vi "Defender.vi"(0 "Field defense":dbl[](array[numeric]), 1 "IA State Input 2":T1, 3 "N atacantes":u32[](array[numeric]), 4 "balls":T4[](array[typedef]), 5 "total de \ndefensores":i32, 6 "geometry":T5, 7 "Defensores":u32[](array[numeric]), 8 "Enemy Robots":T2, 9 "Total de n\natacantes":i32, 10 "Our Robots":T2, 11 "command\nenum":T7) -> (2 "output cluster":T2)   [LabVIEW 2016]
uses:
  Core/AI Robot.ctl
  Functions Enum.ctl
  Command Enum.ctl
  Core/Field Size.ctl
  Core/AI Ball.ctl
  Core/AI Input.ctl
  Core/AI Judge.ctl
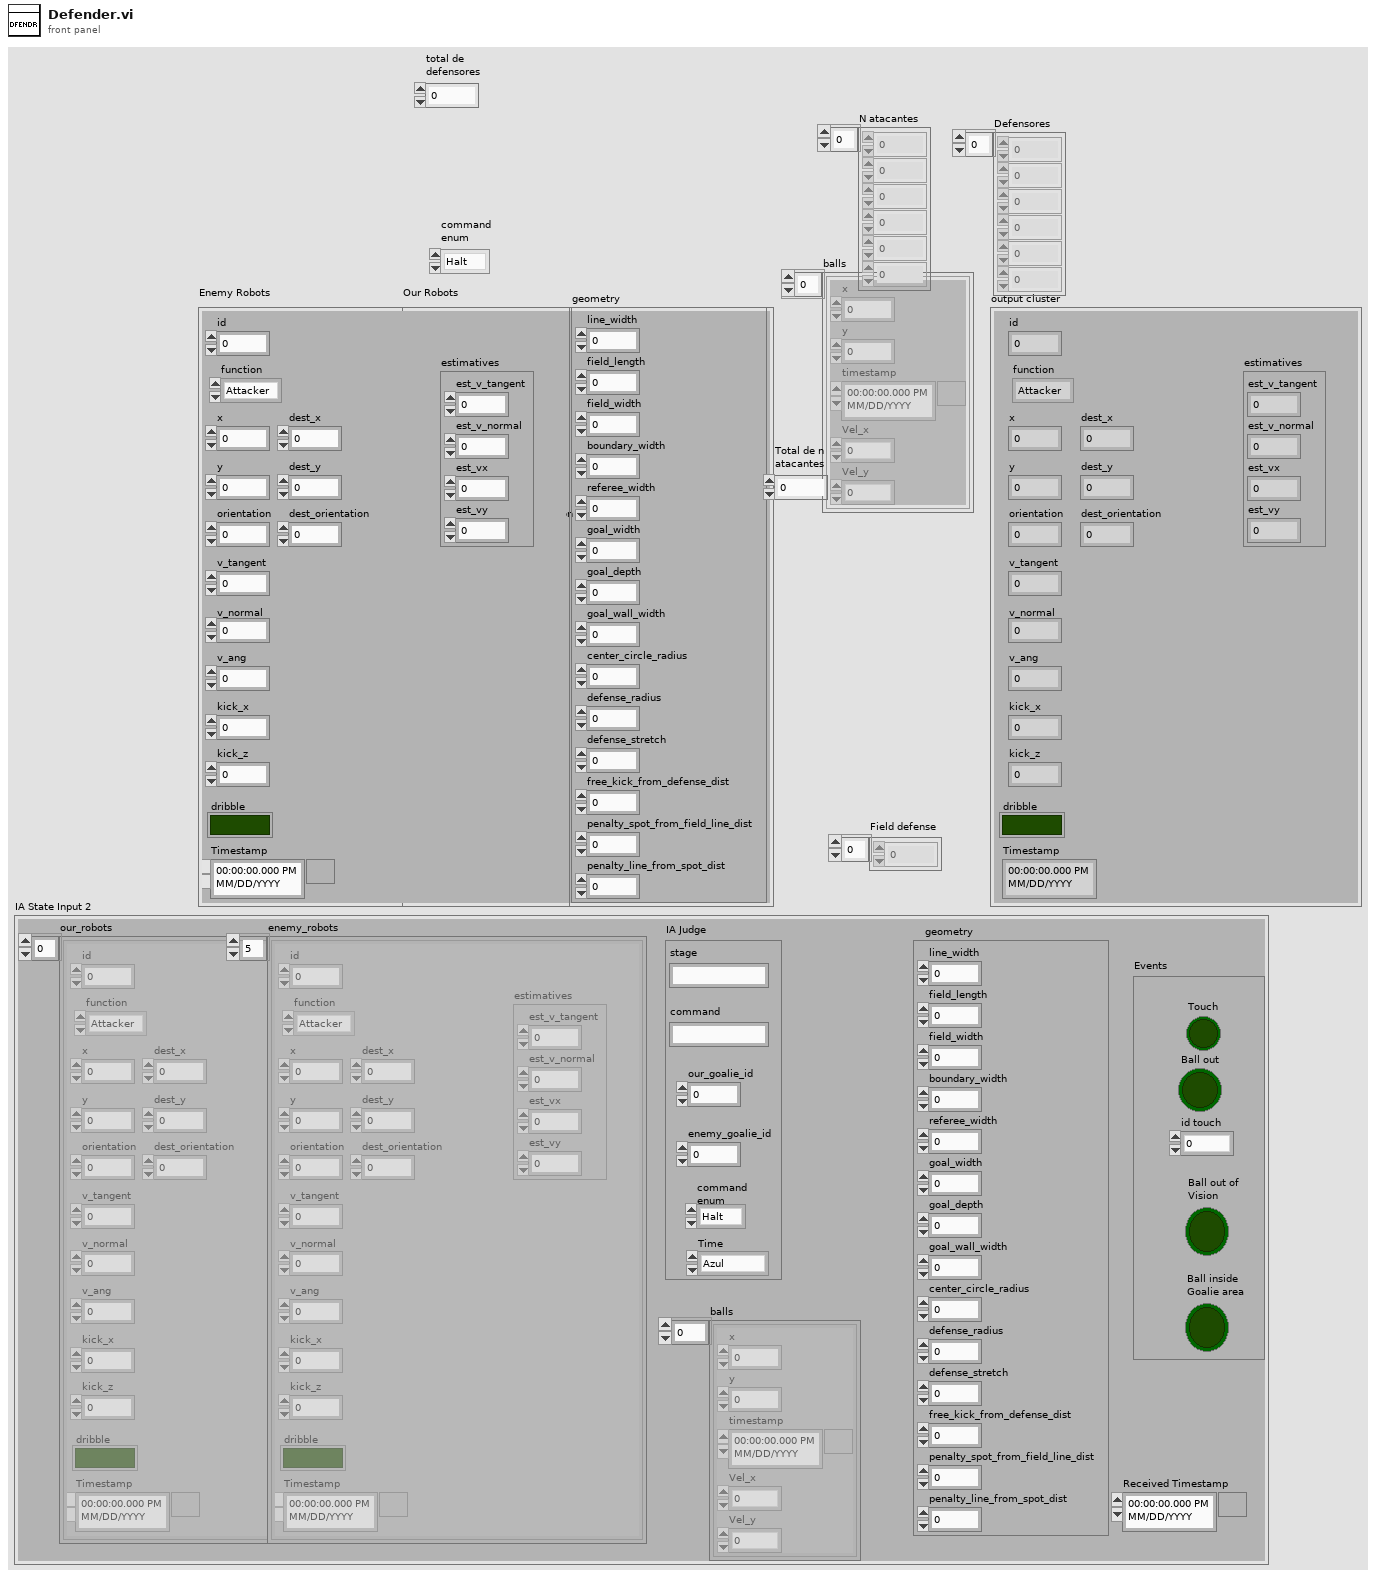
[diagram p1: front panel]
types:
  T1 = typedef "AI Input.ctl" = cluster{"our_robots":T2[], "enemy_robots":T2[], "balls":T4[], "geometry":T5, "IA Judge":T6, "Received Timestamp":timestamp, "Events":cluster{"Touch":bool, "Ball out":bool, "id touch":dbl, "Ball out of \nVision":bool, "Ball inside \nGoalie area":bool}}
  T2 = typedef "AI Robot.ctl" = cluster{"id":u32, "function":T3, "x":dbl, "y":dbl, "orientation":dbl, "v_tangent":dbl, "v_normal":dbl, "v_ang":dbl, "kick_x":dbl, "kick_z":dbl, "dribble":bool, "Timestamp":timestamp, "dest_x":dbl, "dest_y":dbl, "dest_orientation":dbl, "estimatives":cluster{"est_v_tangent":dbl, "est_v_normal":dbl, "est_vx":dbl, "est_vy":dbl}}
  T3 = typedef "Functions Enum.ctl" = enum16{"Attacker", "Goalie", "Defender", "Striker", "Goto 0", "Dummy", "ZigZag"}
  T4 = typedef "AI Ball.ctl" = cluster{"x":dbl, "y":dbl, "timestamp":timestamp, "Vel_x":dbl, "Vel_y":dbl}
  T5 = typedef "Field Size.ctl" = cluster{"line_width":u32, "field_length":u32, "field_width":u32, "boundary_width":u32, "referee_width":u32, "goal_width":u32, "goal_depth":u32, "goal_wall_width":u32, "center_circle_radius":u32, "defense_radius":u32, "defense_stretch":u32, "free_kick_from_defense_dist":u32, "penalty_spot_from_field_line_dist":u32, "penalty_line_from_spot_dist":u32}
  T6 = typedef "AI Judge.ctl" = cluster{"stage":string, "command":string, "our_goalie_id":dbl, "enemy_goalie_id":dbl, "command\nenum":T7, "Time":enum16{"Azul", "Amarelo"}}
  T7 = typedef "Command Enum.ctl" = enum16{"Halt", "Stop", "Force Start", "PKA Normal Start", "Prepare Kickoff Ally", "PKE Normal Start", "Prepare Kickoff Enemy", "Prepare Penalty Ally", "PPA Normal Start", "Prepare Penalty Enemy", "PPE Normal Start", "Direct Free Enemy", "Direct Free Ally", "Indirect Free Enemy", "Indirect Free Ally", "Timeout Enemy", "Timeout Ally", "Goal Enemy", "Goal Ally", "Ball Placement Enemy", "Ball Placement Ally", "None"}
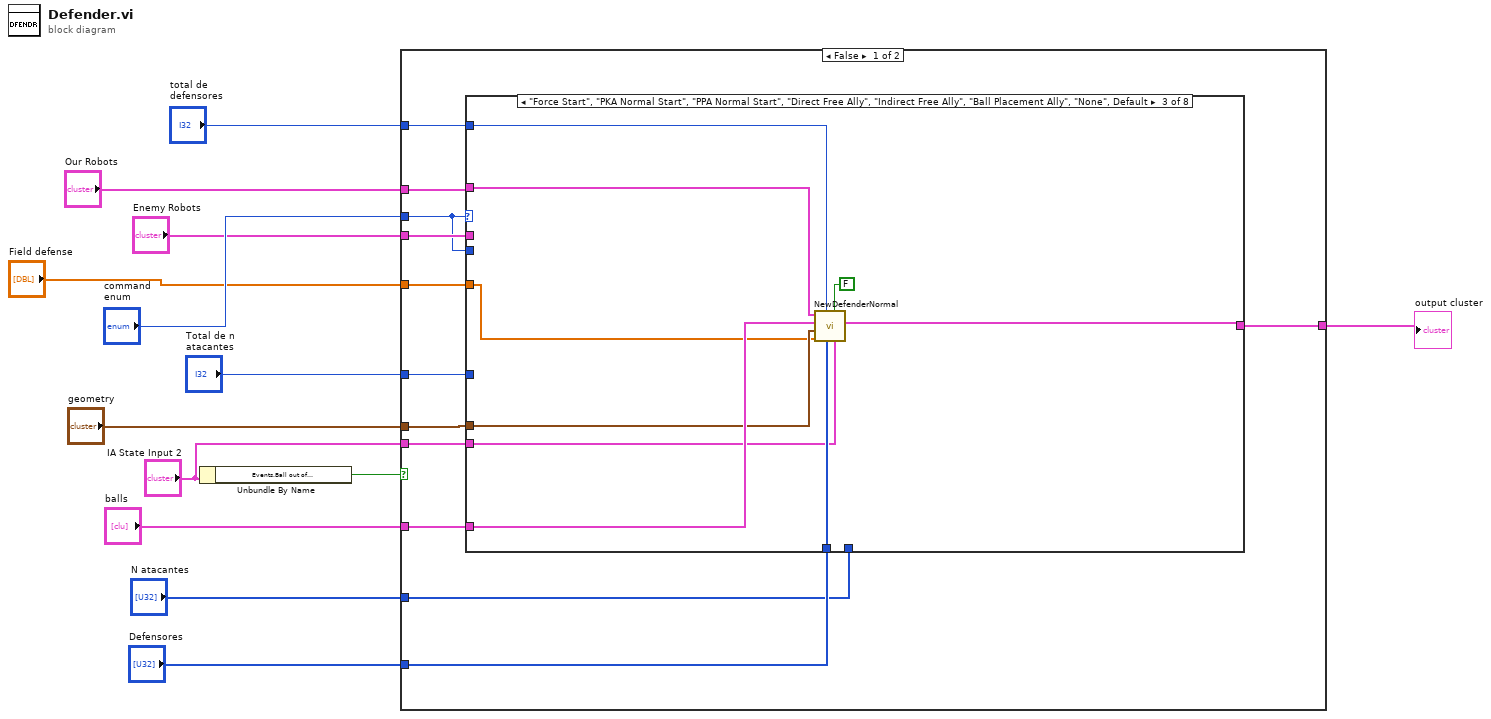
[diagram p0: block diagram]
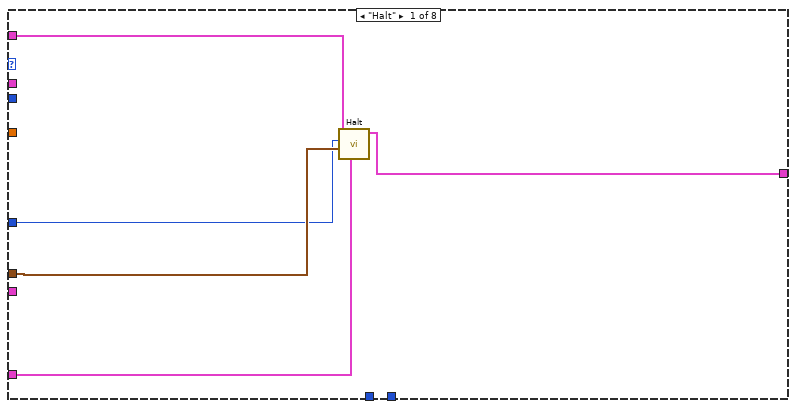
[diagram p2: hidden frame]
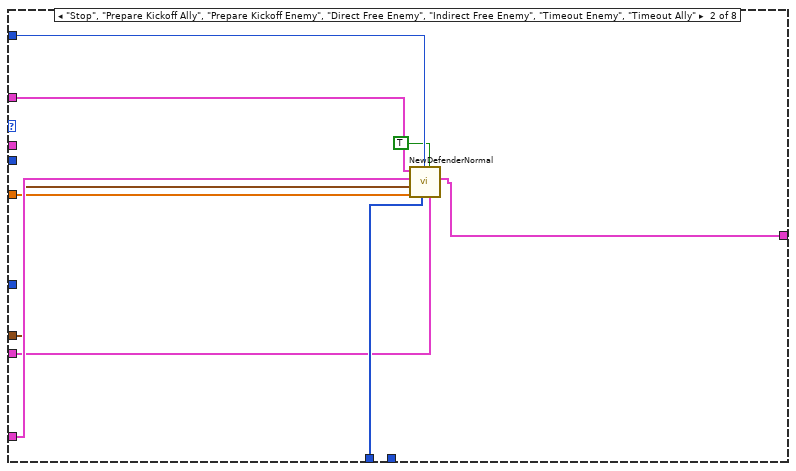
[diagram p3: hidden frame]
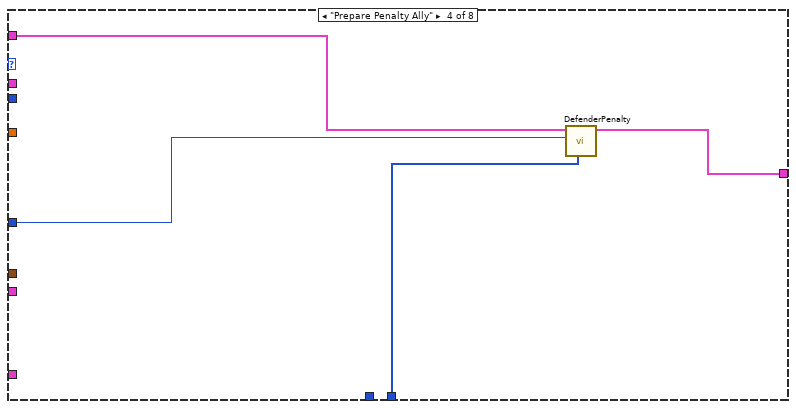
[diagram p4: hidden frame]
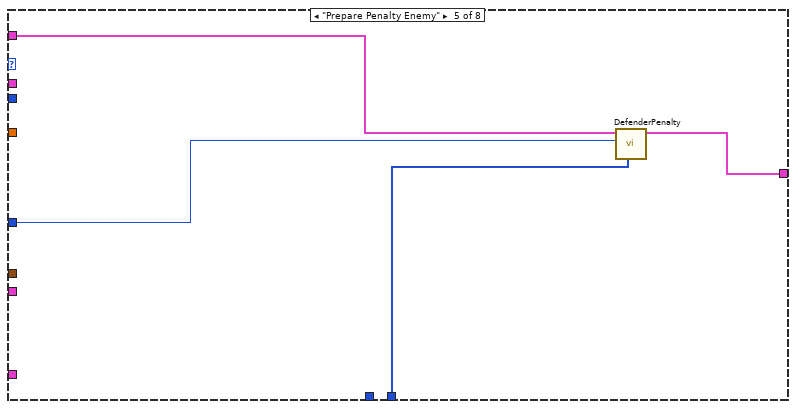
[diagram p5: hidden frame]
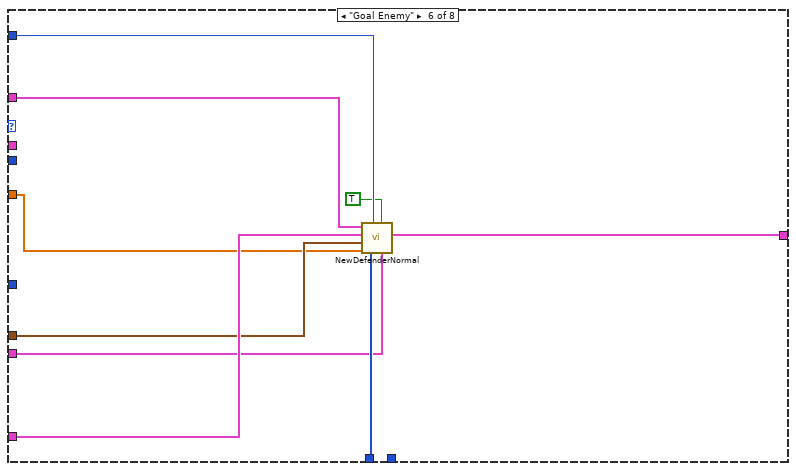
[diagram p6: hidden frame]
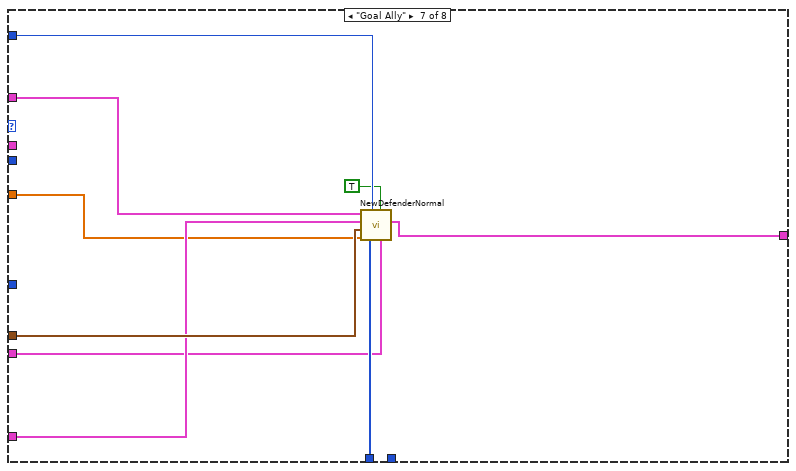
[diagram p7: hidden frame]
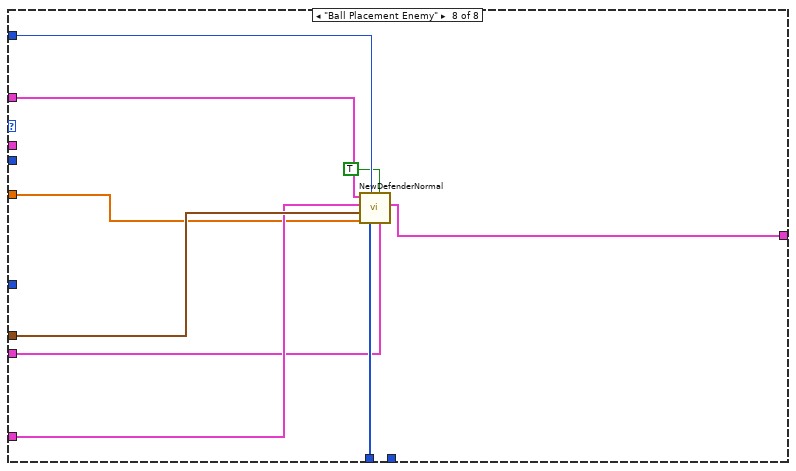
[diagram p8: hidden frame]
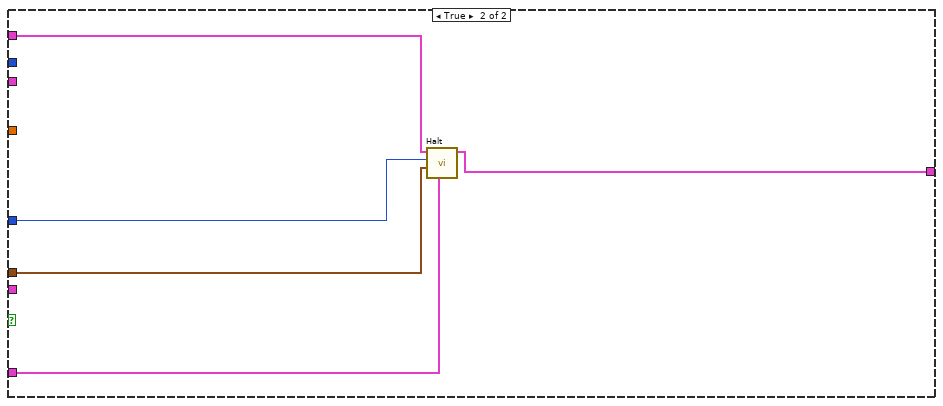
[diagram p9: hidden frame]
diagram:
  n1 = Unbundle By Name("IA State Input 2") -> ("Events.Ball out of \nVision"=w2:bool)
  n2 = case shown="False" w2 {
    tunnel: [w25 w84] -> w13
    tunnel: "Our Robots" -> [w24 w88]
    tunnel: "command\nenum" -> [w14 _]
    tunnel: "balls" -> [w23 w85]
    tunnel: "geometry" -> [w22 w86]
    tunnel: "Total de n\natacantes" -> [w21 w87]
    tunnel: "total de \ndefensores" -> [w20 _]
    tunnel: "Enemy Robots" -> [w19 _]
    tunnel: "Defensores" -> [w18 _]
    tunnel: "N atacantes" -> [w17 _]
    tunnel: "Field defense" -> [w16 _]
    tunnel: "IA State Input 2" -> [w15 _]
    frame False {
      n3 = case shown="\"Force Start\", \"PKA Normal Start\", \"PPA Normal Start\", \"Direct Free Ally\", \"Indirect Free Ally\", \"Ball Placement Ally\", \"None\", Default" w14 {
        tunnel: w24 -> [w26 w37 w47 w52 w56 w64 w71 w80]
        tunnel: [w30 w39 w44 w50 w54 w60 w69 w78] -> w25
        tunnel: w23 -> [w29 w36 w46 _ _ w63 w72 w81]
        tunnel: w22 -> [w28 w35 w45 _ _ w62 w73 w82]
        tunnel: w21 -> [w27 _ _ w51 w55 _ _ _]
        tunnel: w20 -> [_ w38 w48 _ _ w65 w70 w79]
        tunnel: w19 -> [_ _ _ _ _ _ _ _]
        tunnel: w18 -> [_ w34 w43 _ _ w61 w74 w83]
        tunnel: w17 -> [_ _ _ w49 w53 _ _ _]
        tunnel: w16 -> [_ w33 w42 _ _ w59 w68 w77]
        tunnel: w15 -> [_ w32 w41 _ _ w58 w67 w76]
        tunnel: w14 -> [_ _ _ _ _ _ _ _]
        frame "Halt" {
          n4 = call "Halt.vi"("balls"=w29, "Field Size in"=w28, "Numeric"=w27, "Robot in"=w26) -> ("Robot out"=w30:T2)  [unwired: 7 in]
        }
        frame "Stop", "Prepare Kickoff Ally", "Prepare Kickoff Enemy", "Direct Free Enemy", "Indirect Free Enemy", "Timeout Enemy", "Timeout Ally" {
          n5 = call "NewDefenderNormal.vi"("IA State Input 2"=w32, "Stop?"=TRUE, "Defensores"=w34, "total"=w38, "Field defense"=w33, "Field Size in"=w35, "balls"=w36, "Our Robot in"=w37) -> ("Robot out"=w39:T2)  [unwired: 3 in]
        }
        frame "Force Start", "PKA Normal Start", "PPA Normal Start", "Direct Free Ally", "Indirect Free Ally", "Ball Placement Ally", "None", Default {
          n6 = call "NewDefenderNormal.vi"("IA State Input 2"=w41, "Stop?"=FALSE, "Defensores"=w43, "total"=w48, "Field defense"=w42, "Field Size in"=w45, "balls"=w46, "Our Robot in"=w47) -> ("Robot out"=w44:T2)  [unwired: 3 in]
        }
        frame "Prepare Penalty Ally" {
          n7 = call "DefenderPenalty.vi"("N atacantes"=w49, "Total de n \natacantes"=w51, "Robot in"=w52) -> ("Robot out"=w50:T2)  [unwired: 8 in]
        }
        frame "Prepare Penalty Enemy" {
          n8 = call "DefenderPenalty.vi"("N atacantes"=w53, "Total de n \natacantes"=w55, "Robot in"=w56) -> ("Robot out"=w54:T2)  [unwired: 8 in]
        }
        frame "Goal Enemy" {
          n9 = call "NewDefenderNormal.vi"("IA State Input 2"=w58, "Stop?"=TRUE, "Defensores"=w61, "total"=w65, "Field defense"=w59, "Field Size in"=w62, "balls"=w63, "Our Robot in"=w64) -> ("Robot out"=w60:T2)  [unwired: 3 in]
        }
        frame "Goal Ally" {
          n10 = call "NewDefenderNormal.vi"("IA State Input 2"=w67, "Stop?"=TRUE, "Defensores"=w74, "total"=w70, "Field defense"=w68, "Field Size in"=w73, "balls"=w72, "Our Robot in"=w71) -> ("Robot out"=w69:T2)  [unwired: 3 in]
        }
        frame "Ball Placement Enemy" {
          n11 = call "NewDefenderNormal.vi"("IA State Input 2"=w76, "Stop?"=TRUE, "Defensores"=w83, "total"=w79, "Field defense"=w77, "Field Size in"=w82, "balls"=w81, "Our Robot in"=w80) -> ("Robot out"=w78:T2)  [unwired: 3 in]
        }
      }
    }
    frame True {
      n12 = call "Halt.vi"("balls"=w85, "Field Size in"=w86, "Numeric"=w87, "Robot in"=w88) -> ("Robot out"=w84:T2)  [unwired: 7 in]
    }
  }
  "output cluster" <- w13
